vi "PH_TKTDS-30xx.Evt Call Set Display Intensity.vi"(0 "i ref in":refnum<vi>, 1 "Instance":string="N/A", 2 "Display Intensity":u8=1 min=1 max=100 step=1, 5 "error in (no error)":errorcluster) -> (14 "i ref out":refnum<vi>, 19 "error out":errorcluster)   [LabVIEW 2014, in "PH_TKTDS-30xx.lvlib"]
doc: "This VI calls sets a simple call."
uses:
  PH_TKTDS-30xx.lvlib
  CS_Core/CSSystem/CoreLib/CoreLib.short 2 byte array.vi
  CS_Core/CSSystem/CoreLib/CoreLib.lvlib
  CS_Core/BaseProcess/BaseProcess.lvlib
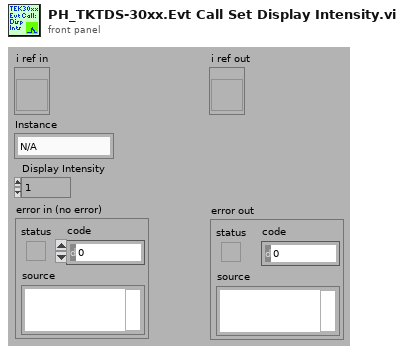
[diagram p1: front panel]
types:
  T1 = typedef "CoreDefs.rawDataType.ctl" = i8[]
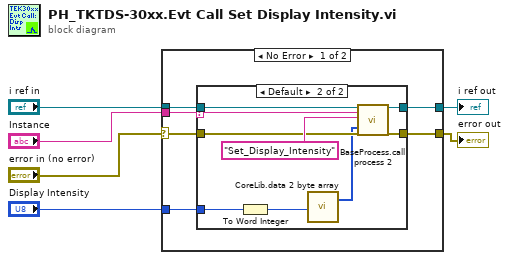
[diagram p0: block diagram]
diagram:
  n1 = case shown="No Error" "error in (no error)" {
    selector: "error in (no error)" -> [w8 w24]
    tunnel: [w12 w25] -> w6
    tunnel: [w11 w24] -> w5
    tunnel: "i ref in" -> [w10 w25]
    tunnel: "Display Intensity" -> [w7 _]
    tunnel: "Instance" -> [w9 _]
    frame No Error {
      n2 = case shown="Default" w9 {
        selector: w9 -> [_ w18]
        tunnel: [w13 w22] -> w12
        tunnel: [w14 w21] -> w11
        tunnel: w10 -> [w13 w20]
        tunnel: w8 -> [w14 w19]
        tunnel: w7 -> [_ w17]
        frame "N/A" {
        }
        frame Default {
          n3 = To Word Integer(number=w17) -> (16bit integer=w15:i16)
          n4 = call-poly "CoreLib.data 2 byte array.vi"("i16"=w15) -> ("byteArray out"=w16:T1)  [unwired: 18 in]
          n5 = call "BaseProcess.call process 2.vi"("i ref in"=w20, "Object"=w18, "Selector"="Set_Display_Intensity", "Data"=w16, "error in (no error)"=w19) -> ("i ref out"=w22:refnum<vi>, "error out"=w21:errorcluster)  [unwired: 13 in]
        }
      }
    }
    frame Error {
    }
  }
  "i ref out" <- w6
  "error out" <- w5
